vi "Wrapper.vi"(8 "error in (no error)":errorcluster, 10 "File Ref":refnum<file>, 11 "Exe Write CRD RDs in":refnum<class "Exe Write CRD RDs.lvclass">) -> (0 "error out":errorcluster, 3 "Exe Write CRD RDs out":refnum<class "Exe Write CRD RDs.lvclass">)   [LabVIEW 2014, in "Controller.lvlib" / "Exe Write CRD RDs.lvclass"]
uses:
  Exe Write CRD RDs.lvclass
  reusable/Data/Data.lvclass
  Instr Exe Write to File/Instr Exe Write to File.lvclass/Instr Exe Write to File.ctl
  reusable/CRDS/Data/Main/CRDS Data.lvclass
  reusable/CRDS/Data/Cell/CRDS Cell Data.lvclass/CRDS Cell Data.ctl
  reusable/CRDS/Data/Cell/Read Laser Data.vi
  Instr Exe Write to File/Read MAP DVR.vi
  Instr Exe Write to File/Read DataObj.vi
  reusable/Data/Read measTime.vi
  reusable/CRDS/Data/Main/Read CellData.vi
  reusable/CRDS/Data/Cell/CRDS Cell Data.lvclass
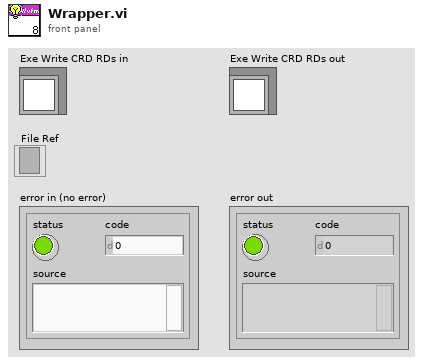
[diagram p1: front panel]
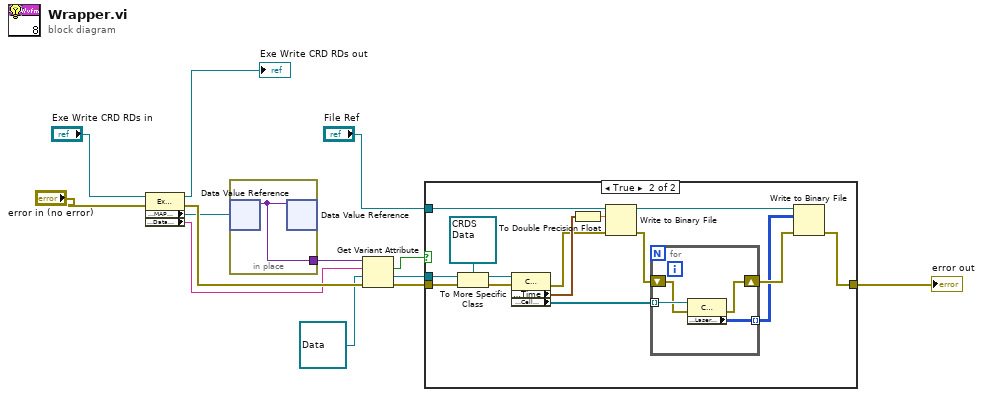
[diagram p0: block diagram]
diagram:
  n1 = property class="Exe Write CRD RDs"(reference="Exe Write CRD RDs in", error in="error in (no error)") -> (reference out=→"Exe Write CRD RDs out":refnum<class "Exe Write CRD RDs.lvclass">, error out=w8:errorcluster, "Accessors:MAP DVR"=w5:refnum<data-value>, "Accessors:DataObj"=w6:string)
  n2 = in-place {
    in-place-border: [w14] -> w1
    n3 = in-place-dvr #1(w5) -> (w14:variant)  [unwired: 1 out]
    n4 = in-place-dvr #1(w14) -> ()  [unwired: 2 out]
  }
  n5 = Get Variant Attribute(Variant=w1, name=w6, default value (empty Variant)=refnum<class "Data.lvclass"> refnum ("Base Data Lib:Data"), error in=w8) -> (found=w3:bool, value=w2:refnum<class "Data.lvclass">, error out=w4:errorcluster)  [unwired: 1 out]
  n6 = case shown="True" w3 {
    tunnel: [w15 w17] -> w13
    tunnel: "File Ref" -> [_ w25]
    tunnel: w2 -> [_ w30]
    tunnel: w4 -> [w15 w23]
    frame False {
    }
    frame True {
      n7 = To More Specific Class(target class=refnum<class "CRDS Data.lvclass"> refnum ("CRDS Lib.lvlib:CRDS"), reference=w30, error in=w23) -> (specific class reference=w29:refnum<class "CRDS Data.lvclass">, error out=w22:errorcluster)
      n8 = property class="CRDS"(reference=w29, error in=w22) -> (error out=w21:errorcluster, "Accessors:Time"=w27:timestamp, "Accessors:Cell Data"=w28:refnum<class "CRDS Cell Data.lvclass">[])  [unwired: 1 out]
      n9 = To Double Precision Float(number=w27) -> (double precision float=w26:dbl)
      n10 = Write to Binary File(file (use dialog)=w25, data=w26, error in=w21) -> (refnum out=w19:refnum<file>, error out=w24:errorcluster)  [unwired: 3 in, 1 out]
      n11 = for {
        tunnel: w28 -> [w34] mode=indexing
        shift-right: [w32] -> w20
        shift-left: w24 -> [w33]
        tunnel: [w31] -> w18 mode=indexing
        n12 = property class="CRDS Cell"(reference=w34, error in=w33) -> (error out=w32:errorcluster, "Accessors:Laser Data"=w31:i16[][])  [unwired: 1 out]
      }
      n13 = Write to Binary File(file (use dialog)=w19, data=w18, error in=w20) -> (error out=w17:errorcluster)  [unwired: 3 in, 2 out]
    }
  }
  "error out" <- w13
